vi "read_timing_array.vi"(4 "error in":errorcluster, 5 "input array":dbl[](array[numeric]), 7 "VISA resource in":refnum<visa-resource-name>) -> (0 "error out 2":errorcluster, 1 "delay array":dbl[](array[numeric]), 3 "VISA resource out":refnum<visa-resource-name>)   [LabVIEW 2011]
doc: "Reads all delay values stored in the DG645 and returns them in an array, from t0 to H.\nSee DG645 documentation for mor info."
panel:
  in  "bytes to read":u32=256
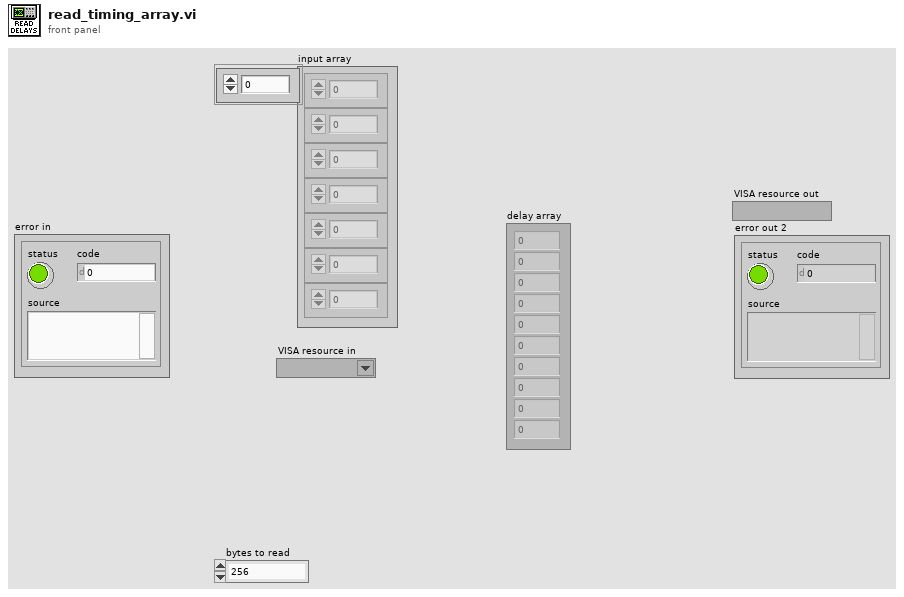
[diagram p1: front panel]
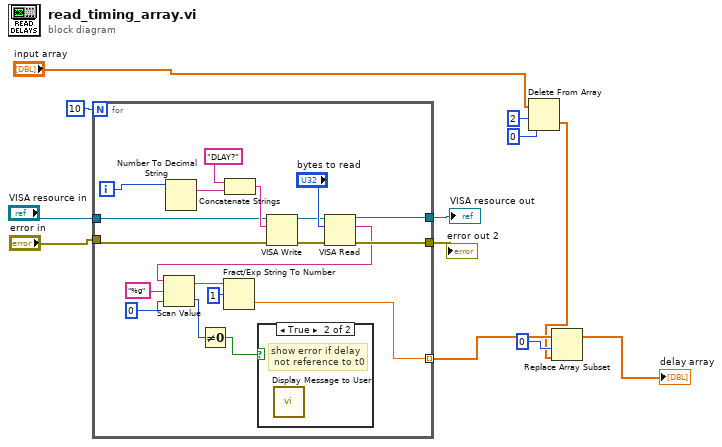
[diagram p0: block diagram]
diagram:
  n1 = for {
    N: 10 -> [_]
    tunnel: "error in" -> [w28]
    tunnel: [w25] -> w5 mode=indexing
    tunnel: [w22] -> w8
    tunnel: "VISA resource in" -> [w17]
    tunnel: [w16] -> w9
    i -> [w13]
    n2 = Number To Decimal String(number=w13) -> (decimal integer string=w24:string)  [unwired: 1 in]
    n3 = Concatenate Strings("DLAY?" ("string"), w24) -> (w23:string)
    n4 = VISA Write(VISA resource name=w17, write buffer=w23, error in (no error)=w28) -> (VISA resource name out=w30:refnum<visa-resource-name>, error out=w29:errorcluster)  [unwired: 1 out]
    n5 = VISA Read(VISA resource name=w30, byte count="bytes to read", error in (no error)=w29) -> (VISA resource name out=w16:refnum<visa-resource-name>, read buffer=w15:string, error out=w22:errorcluster)  [unwired: 1 out]
    n6 = Scan Value(string=w15, format string="%g", default (0 dbl)=u16 0) -> (output string=w19:string, value=w18:u16)
    n7 = Not Equal To 0?(x=w18) -> (x != 0?=w14:bool)
    n8 = Fract/Exp String To Number(string=w19, offset=1) -> (number=w25:dbl)  [unwired: 2 in, 1 out]
    n9 = case shown="True" w14 {
      frame False {
      }
      frame True {
        # "show error if delay\n not reference to t0"
        n10 = call "Display Message to User"() -> ()  [unwired: 10 in, 2 out]
      }
    }
  }
  "VISA resource out" <- w9
  "error out 2" <- w8
  n11 = Delete From Array(array="input array", length=2, index=0) -> (deleted portion=w2:dbl[])  [unwired: 1 out]
  n12 = Replace Array Subset(array=w5, new element=w2, index=0) -> (→"delay array":dbl[])
